vi "for_simple.vi"() -> ()   [LabVIEW 2021]
uses:
  <vilib>/numeric/Random Number (Range) DBL.vi
panel:
  out "Boolean":bool
  out "random number":dbl
  out "iteration counter":i32
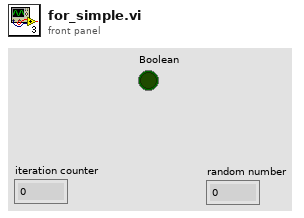
[diagram p1: front panel]
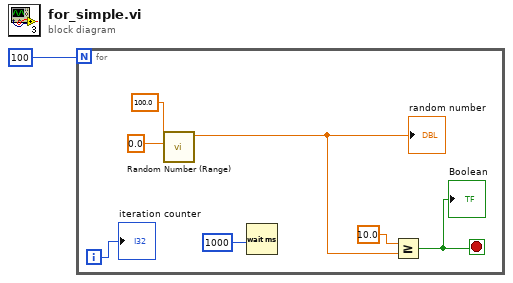
[diagram p0: block diagram]
diagram:
  n1 = for {
    N: 100 -> [_]
    i -> [w6]
    stop <- w2 stop-if-true
    n2 = call-poly <vilib>:"Random Number (Range).vi"("lower bound (0)"=0.0, "upper bound (100)"=100.0) -> ("number"=w4:dbl)  [unwired: 9 in]
    "random number" <- w4
    n3 = Wait (ms)(milliseconds to wait=1000) -> ()  [unwired: 1 out]
    n4 = Greater Or Equal?(x=10.0, y=w4) -> (x >= y?=w2:bool)
    "Boolean" <- w2
    "iteration counter" <- w6
  }
